vi "VISA Write.vi"(8 "error in":errorcluster, 10 "SCPI command":string, 11 "VISA resource in":refnum<visa-resource-name>) -> (0 "error out":errorcluster, 2 "Bytes at Port out":u32, 3 "VISA resource out":refnum<visa-resource-name>)   [LabVIEW 2021, in "Keysight U1282A.lvlib"]
doc: "Este VI permite escribir un comando SCIP mediante puerto serial VISA con los tiempos de espera requeridos por el instrumento U1282A"
uses:
  Keysight U1282A.lvlib
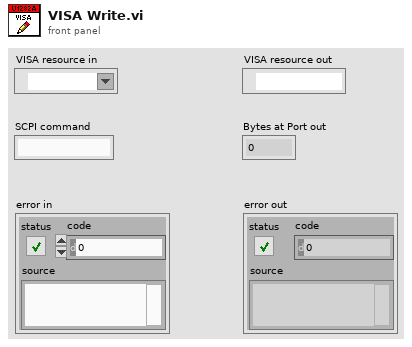
[diagram p1: front panel]
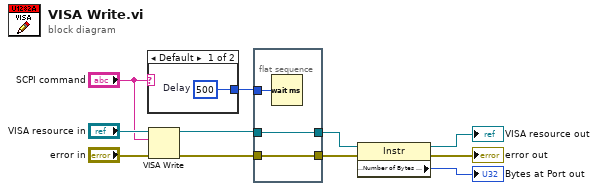
[diagram p0: block diagram]
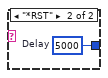
[diagram p2: hidden frame]
diagram:
  n1 = case shown="Default" "SCPI command" {
    tunnel: [w12 w13] -> w9
    frame Default {
      w12 = u32 500  # Delay
    }
    frame "*RST" {
      w13 = u32 5000  # Delay
    }
  }
  n2 = VISA Write(VISA resource name="VISA resource in", write buffer="SCPI command", error in (no error)="error in") -> (VISA resource name out=w11:refnum<visa-resource-name>, error out=w2:errorcluster)  [unwired: 1 out]
  n3 = flat-sequence {
    tunnel: [w14] -> w1
    tunnel: [w16] -> w10
    tunnel: w11 -> [w16]
    tunnel: w9 -> [w15]
    tunnel: w2 -> [w14]
    frame #0 {
      n4 = Wait (ms)(milliseconds to wait=w15) -> ()  [unwired: 1 out]
    }
  }
  n5 = property class="Instr"(reference=w10, error in=w1) -> (reference out=→"VISA resource out":refnum<visa-resource-name>, error out=→"error out":errorcluster, "Serial Settings:Number of Bytes at Serial Port"=→"Bytes at Port out":u32)
